vi "16TMonitor.vi"() -> ()   [LabVIEW 2016]
uses:
  Utility/Monitor Communication/S16/16T-Cluster.ctl
  Global/Global Variables/Data_Display_global.vi
  Instrument_Setup.vi
  Utility/Monitor Communication/sub-vis/16T_Open_Queue.vi
  Utility/Monitor Communication/sub-vis/16T_Check_Queue.vi
panel:
  out "16 T Cluster":T1={"Clamp"=FALSE, "Switch Heater"=FALSE, "Go to Zero"=FALSE, "Go to set"=FALSE, "Go to Hold"=FALSE, "Clamped"=FALSE, "Quenched"=FALSE, "Rate limit"=FALSE, "Persistent"=FALSE, "Hold"=FALSE, "Set"=FALSE, "Zero"=FALSE, "Magnet (T)"=0.0, "Leads (T)"=0.0, "Magnet T (K)"=3.4572, "Switch"=FALSE, "Setpoint (T)"=3.4572, "Rate (T/min)"=0.0, "Select"=FALSE, "Sweeping"=FALSE} {"Rate (T/min)" format="%6_5f"; "Setpoint (T)" format="%6_5f"; "Magnet T (K)" format="%6_5f"}
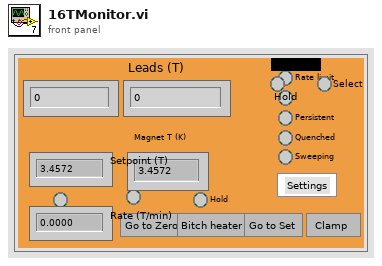
[diagram p1: front panel]
types:
  T1 = typedef "16T-Cluster.ctl" = cluster{"Clamp":bool, "Switch Heater":bool, "Go to Zero":bool, "Go to set":bool, "Go to Hold":bool, "Clamped":bool, "Quenched":bool, "Rate limit":bool, "Persistent":bool, "Hold":bool, "Set":bool, "Zero":bool, "Magnet (T)":dbl, "Leads (T)":dbl, "Magnet T (K)":dbl, "Switch":bool, "Setpoint (T)":dbl, "Rate (T/min)":dbl, "Select":bool, "Sweeping":bool}
  T2 = typedef "PSIO.ctl" = cluster{"Address":T3, "Version":enum16{"PS", "IPS"}}
  T3 = typedef "OxfordAddress.ctl" = cluster{"Com Port":i32, "ISOBUS Address":i32, "GPIB Address":i16, "Communication":enum16{"RS232", "ISOBUS", "GPIB", "Gateway"}}
  T4 = cluster{"Version\n":string, "Max Sweep(4.2K)":dbl[unit], "Max Sweep(2.2K)":dbl[unit], "Switch htr dly":dbl[unit], "Max Field(4.2K)":dbl[unit], "Max Field(2.2K)":dbl[unit], "Max lead res":dbl[unit], "IO Info":T2}
  T5 = cluster{"Max 4.2K temp":dbl[unit], "Max 2.2K temp":dbl[unit], "Instrument address":cluster{"Com Port":i32, "ISOBUS Address":i32, "GPIB Address":i16, "Communication":enum16{"RS232", "ISOBUS", "GPIB", "Gateway"}}}
  T6 = cluster{"Com Port":i32, "ISOBUS Address":i32, "GPIB Address":i16, "Communication":enum16{"RS232", "ISOBUS", "GPIB", "Gateway"}}
  T7 = cluster{"Value":i16, "At rest":bool, "Sweeping":bool, "Rate limiting":bool}
  T8 = cluster{"Value":i16, "Hold":bool, "To set point":bool, "To zero":bool, "Clamped":bool}
  T9 = cluster{"Value":i16, "Off (at zero field)":bool, "On":bool, "Off (at field)":bool, "No switch fitted":bool, "Confirm":bool}
  T10 = cluster{"Value":i16, "Desired":u16, "Magnet":u16, "Commanded":u16, "Actual":u16}
  T11 = cluster{"Value":i16, "Quenched":bool, "Over heated":bool, "Warming up":bool}
  T12 = typedef "16T_Control.ctl" = cluster{"Clamp":bool, "Switch Heater":bool, "Go to Zero":bool, "Go to Set":bool, "Go to Hold":bool, "Setpoint (T)":dbl, "Rate (T/min)":dbl, "Set Rate":bool}
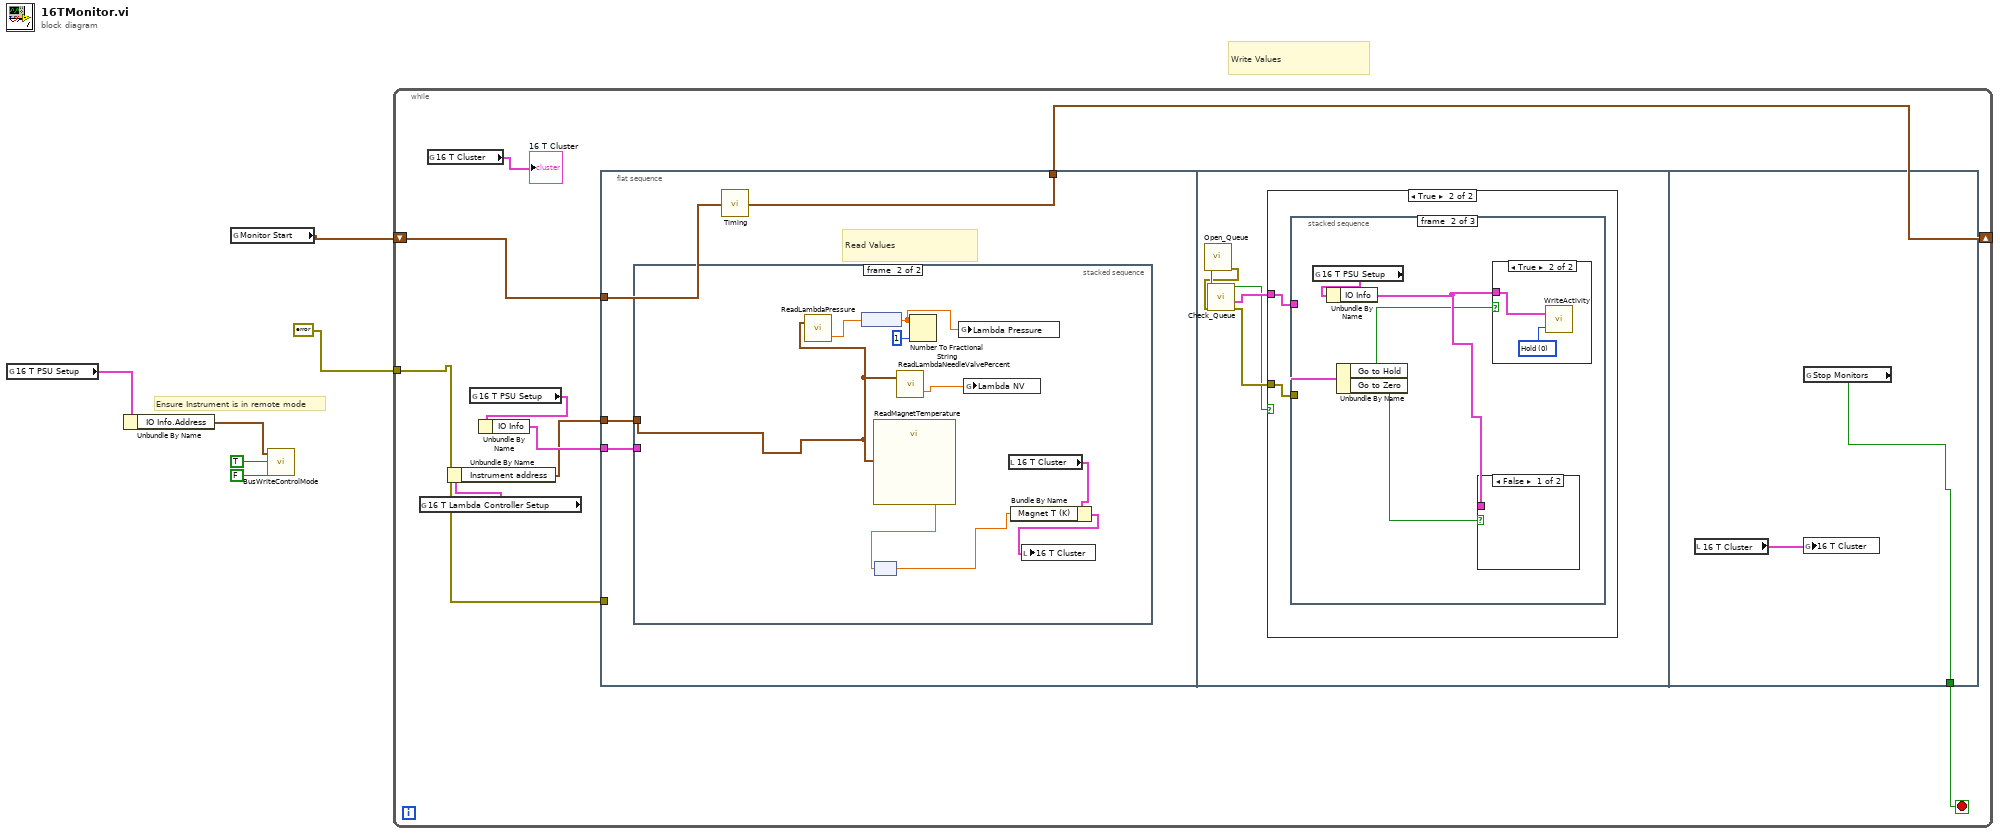
[diagram p0: block diagram]
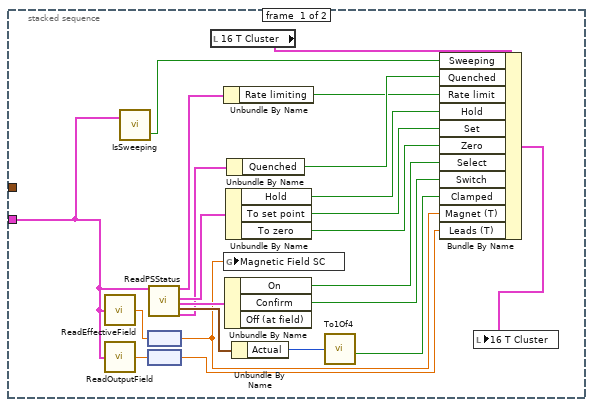
[diagram p2: hidden frame]
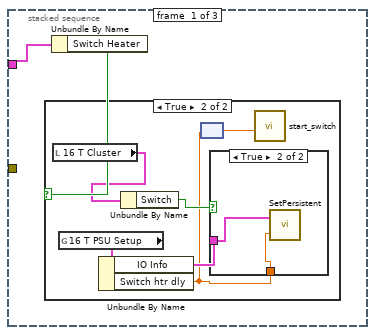
[diagram p4: hidden frame]
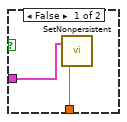
[diagram p6: hidden frame]
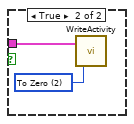
[diagram p7: hidden frame]
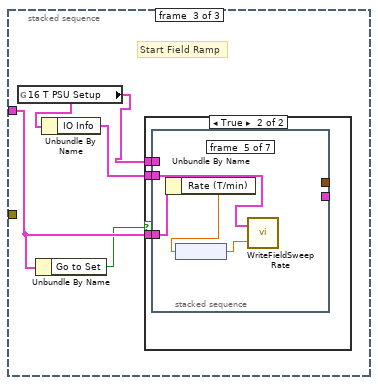
[diagram p9: hidden frame]
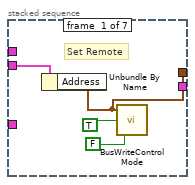
[diagram p11: hidden frame]
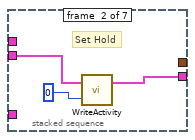
[diagram p12: hidden frame]
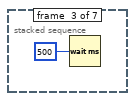
[diagram p13: hidden frame]
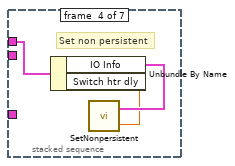
[diagram p14: hidden frame]
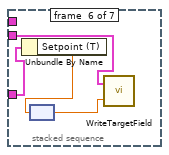
[diagram p15: hidden frame]
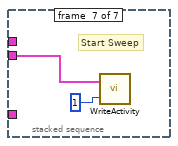
[diagram p16: hidden frame]
diagram:
  # "Ensure Instrument is in remote mode"
  # "Write Values"
  n1 = global read "Instrument_Setup.vi" "16 T PSU Setup"() -> (w4:T4)
  n2 = Unbundle By Name(w4) -> ("IO Info.Address"=w3:T3)
  n3 = global read "Data_Display_global.vi" "Monitor Start"() -> (w6:timestamp)
  n4 = call "BusWriteControlMode.vi"("Locked"=FALSE, "Remote"=TRUE, "Address"=w3) -> ()  [unwired: 1 out]
  n5 = while {
    tunnel: errorcluster {"status"=FALSE, "code"=0, "source"=""} ("error constant") -> [w15]
    shift-right: [w13] -> _
    shift-left: w6 -> [w14]
    stop <- w11 stop-if-true
    n6 = global read "Instrument_Setup.vi" "16 T Lambda Controller Setup"() -> (w8:T5)
    n7 = global read "Data_Display_global.vi" "16 T Cluster"() -> (→"16 T Cluster":T1)
    n8 = Unbundle By Name(w8) -> ("Instrument address"=w7:T6)
    n9 = global read "Instrument_Setup.vi" "16 T PSU Setup"() -> (w9:T4)
    n10 = Unbundle By Name(w9) -> ("IO Info"=w10:T2)
    n11 = flat-sequence {
      tunnel: w15 -> [_]
      tunnel: w14 -> [w18]
      tunnel: [w19] -> w13
      tunnel: w10 -> [w17]
      tunnel: w7 -> [w16]
      tunnel: [w107] -> w11
      frame #0 {
        # "Read Values"
        n12 = stacked-sequence {
          tunnel: w16 -> [_ w45]
          tunnel: w17 -> [w21 _]
          frame #0 {
            n13 = call "ReadEffectiveField.vi"("IO Info"=w21) -> ("Effective field"=w25:dbl[unit])  [unwired: 2 out]
            n14 = call "ReadOutputField.vi"("IO Info"=w21) -> ("Field"=w27:dbl[unit])  [unwired: 2 out]
            n15 = call "IsSweeping.vi"("IO Info"=w21) -> ("Sweeping"=w20:bool)  [unwired: 1 in, 1 out]
            n16 = node(w25) -> (w24:dbl)
            n17 = node(w27) -> (w26:dbl)
            n18 = call "ReadPSStatus.vi"("IO Info"=w21) -> ("Mode (n)"=w39:T7, "Activity"=w40:T8, "Switch Heater"=w38:T9, "Polarity"=w37:T10, "System Status (m)"=w36:T11)  [unwired: 10 in, 4 out]
            n19 = local read "16 T Cluster"() -> (w22:T1)
            n20 = Unbundle By Name(w39) -> ("Rate limiting"=w33:bool)
            n21 = global write "Data_Display_global.vi" "Magnetic Field SC"(w24) -> ()
            n22 = Unbundle By Name(w38) -> ("On"=w29:bool, "Confirm"=w28:bool)  [unwired: 1 out]
            n23 = Unbundle By Name(w40) -> ("Hold"=w32:bool, "To set point"=w31:bool, "To zero"=w30:bool)
            n24 = Unbundle By Name(w36) -> ("Quenched"=w34:bool)
            n25 = Unbundle By Name(w37) -> ("Actual"=w41:u16)
            n26 = call "To1Of4.vi"("Input"=w41) -> ("3"=w35:bool)  [unwired: 3 out]
            n27 = Bundle By Name(cluster=w22, "Sweeping"=w20, "Quenched"=w34, "Rate limit"=w33, "Hold"=w32, "Set"=w31, "Zero"=w30, "Select"=w29, "Switch"=w28, "Clamped"=w35, "Magnet (T)"=w24, "Leads (T)"=w26) -> (w23:T1)
            n28 = local write "16 T Cluster"(w23) -> ()
          }
          frame #1 {
            n29 = call "ReadLambdaPressure.vi"("Address"=w45) -> ("Pressure"=w48:dbl[unit])  [unwired: 1 in, 1 out]
            n30 = node(w48) -> (w46:dbl)
            n31 = call "ReadMagnetTemperature.vi"("Address"=w45) -> ("Magnet Temperature"=w50:dbl[unit])  [unwired: 1 in, 1 out]
            n32 = node(w50) -> (w44:dbl)
            n33 = call "ReadLambdaNeedleValvePercent.vi"("Address"=w45) -> ("Actual Needle Valve  %"=w47:dbl)  [unwired: 1 in, 1 out]
            n34 = Number To Fractional String(number=w46, precision (6)=1) -> ()  [unwired: 2 in, 1 out]
            n35 = global write "Data_Display_global.vi" "Lambda Pressure"(w46) -> ()
            n36 = global write "Data_Display_global.vi" "Lambda NV"(w47) -> ()
            n37 = local read "16 T Cluster"() -> (w43:T1)
            n38 = Bundle By Name(cluster=w43, "Magnet T (K)"=w44) -> (w42:T1)
            n39 = local write "16 T Cluster"(w42) -> ()
          }
        }
        n40 = call "Timing.vi"("start time (s)"=w18) -> ("last reading (s)"=w19:timestamp)
      }
      frame #1 {
        n41 = call-poly "Open_Queue.vi"() -> ("error out"=w54:errorcluster, "queue out"=w55:refnum<queue>)  [unwired: 10 in]
        n42 = call-poly "Check_Queue.vi"("error in (no error)"=w54, "queue"=w55) -> ("error out"=w53:errorcluster, "16 T Magnet control"=w52:T12, "New Entries?"=w51:bool)  [unwired: 6 in]
        n43 = case shown="True" w51 {
          tunnel: w53 -> [_ w57]
          tunnel: w52 -> [_ w56]
          frame False {
          }
          frame True {
            n44 = stacked-sequence {
              tunnel: w57 -> [_ _ _]
              tunnel: w56 -> [w59 w72 w80]
              frame #0 {
                n45 = Unbundle By Name(w59) -> ("Switch Heater"=w58:bool)
                n46 = case shown="True" w58 {
                  frame False {
                  }
                  frame True {
                    n47 = local read "16 T Cluster"() -> (w65:T1)
                    n48 = global read "Instrument_Setup.vi" "16 T PSU Setup"() -> (w63:T4)
                    n49 = Unbundle By Name(w63) -> ("IO Info"=w62:T2, "Switch htr dly"=w61:dbl[unit])
                    n50 = Unbundle By Name(w65) -> ("Switch"=w64:bool)
                    n51 = node(w61) -> (w60:dbl)
                    n52 = case shown="True" w64 {
                      tunnel: w62 -> [w67 w69]
                      tunnel: w61 -> [w66 w68]
                      frame False {
                        n53 = call "SetNonpersistent.vi"("Switch Heater Dwell Time"=w66, "IO Info"=w67) -> ()  [unwired: 2 out]
                      }
                      frame True {
                        n54 = call "SetPersistent.vi"("Switch Heater Dwell Time"=w68, "IO Info"=w69) -> ()  [unwired: 1 in, 1 out]
                      }
                    }
                    n55 = call "start_switch.vi"("Switch heater time"=w60) -> ()  [unwired: 2 in]
                  }
                }
              }
              frame #1 {
                n56 = global read "Instrument_Setup.vi" "16 T PSU Setup"() -> (w74:T4)
                n57 = Unbundle By Name(w74) -> ("IO Info"=w73:T2)
                n58 = Unbundle By Name(w72) -> ("Go to Hold"=w71:bool, "Go to Zero"=w70:bool)
                n59 = case shown="False" w70 {
                  tunnel: w73 -> [_ w76]
                  frame False {
                  }
                  frame True {
                    w75 = u16 2 items=["Hold", "To Set Point", "To Zero", "Clamp"] ("Activity")
                    n60 = call "WriteActivity.vi"("Activity"=w75, "IO Info"=w76) -> ()  [unwired: 1 in, 1 out]
                  }
                }
                n61 = case shown="True" w71 {
                  tunnel: w73 -> [_ w78]
                  frame False {
                  }
                  frame True {
                    w77 = u16 0 items=["Hold", "To Set Point", "To Zero", "Clamp"] ("Activity")
                    n62 = call "WriteActivity.vi"("Activity"=w77, "IO Info"=w78) -> ()  [unwired: 1 in, 1 out]
                  }
                }
              }
              frame #2 {
                # "Start Field Ramp"
                n63 = global read "Instrument_Setup.vi" "16 T PSU Setup"() -> (w81:T4)
                n64 = Unbundle By Name(w80) -> ("Go to Set"=w79:bool)
                n65 = Unbundle By Name(w81) -> ("IO Info"=w82:T2)
                n66 = case shown="True" w79 {
                  tunnel: w82 -> [_ w85]
                  tunnel: w81 -> [_ w84]
                  tunnel: w80 -> [_ w83]
                  frame False {
                  }
                  frame True {
                    n67 = stacked-sequence {
                      tunnel: [_ w92 _ _ _ _ _] -> _
                      tunnel: w85 -> [w87 w90 _ _ w99 w101 w105]
                      tunnel: [w86 _ _ _ _ _ _] -> _
                      tunnel: w84 -> [_ _ _ w94 _ _ _]
                      tunnel: w83 -> [_ _ _ _ w100 w104 _]
                      frame #0 {
                        # "Set Remote"
                        n68 = Unbundle By Name(w87) -> ("Address"=w86:T3)
                        n69 = call "BusWriteControlMode.vi"("Locked"=FALSE, "Remote"=TRUE, "Address"=w86) -> ()  [unwired: 1 out]
                      }
                      frame #1 {
                        # "Set Hold"
                        n70 = call "WriteActivity.vi"("Activity"=0, "IO Info"=w90) -> ("IO Info"=w92:T2)  [unwired: 1 in]
                      }
                      frame #2 {
                        n71 = Wait (ms)(milliseconds to wait=u32 500) -> ()  [unwired: 1 out]
                      }
                      frame #3 {
                        # "Set non persistent"
                        n72 = Unbundle By Name(w94) -> ("IO Info"=w96:T2, "Switch htr dly"=w95:dbl[unit])
                        n73 = call "SetNonpersistent.vi"("Switch Heater Dwell Time"=w95, "IO Info"=w96) -> ()  [unwired: 2 out]
                      }
                      frame #4 {
                        n74 = Unbundle By Name(w100) -> ("Rate (T/min)"=w98:dbl)
                        n75 = node(w98) -> (w97:dbl[unit])
                        n76 = call "WriteFieldSweepRate.vi"("Sweep rate"=w97, "IO Info"=w99) -> ()  [unwired: 1 out]
                      }
                      frame #5 {
                        n77 = Unbundle By Name(w104) -> ("Setpoint (T)"=w103:dbl)
                        n78 = node(w103) -> (w102:dbl[unit])
                        n79 = call "WriteTargetField.vi"("Target Field"=w102, "IO Info"=w101) -> ()  [unwired: 1 in, 1 out]
                      }
                      frame #6 {
                        # "Start Sweep"
                        n80 = call "WriteActivity.vi"("Activity"=1, "IO Info"=w105) -> ()  [unwired: 1 in, 1 out]
                      }
                    }
                  }
                }
              }
            }
          }
        }
      }
      frame #2 {
        n81 = local read "16 T Cluster"() -> (w108:T1)
        n82 = global write "Data_Display_global.vi" "16 T Cluster"(w108) -> ()
        n83 = global read "Data_Display_global.vi" "Stop Monitors"() -> (w107:bool)
      }
    }
  }
